vi "set 6221 level(SubVI).vi"(8 "错误输入（无错误）":errorcluster, 10 "电流（mA）":dbl, 11 "VISA引用句柄输入":refnum<visa-resource-name>) -> (0 "错误输出":errorcluster, 3 "VISA引用句柄输出":refnum<visa-resource-name>)   [LabVIEW 2019, in "SubVI.lvlib"]
uses:
  SubVI.lvlib
  lib/Keithley 622x/Configure/Delta PDelta DCon Modes/Low Level/Typedefs/KE622x -- Delta PDelta Mode High Level.ctl
  lib/Keithley 622x/Keithley 622x.lvlib
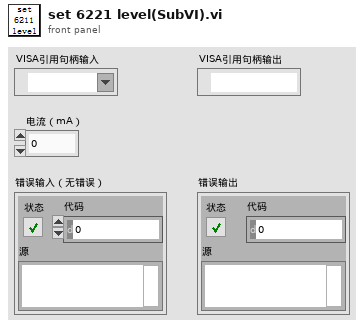
[diagram p1: front panel]
types:
  T1 = typedef "Keithley 622x.lvlib/KE622x -- Delta PDelta Mode High Level.ctl" = dbl
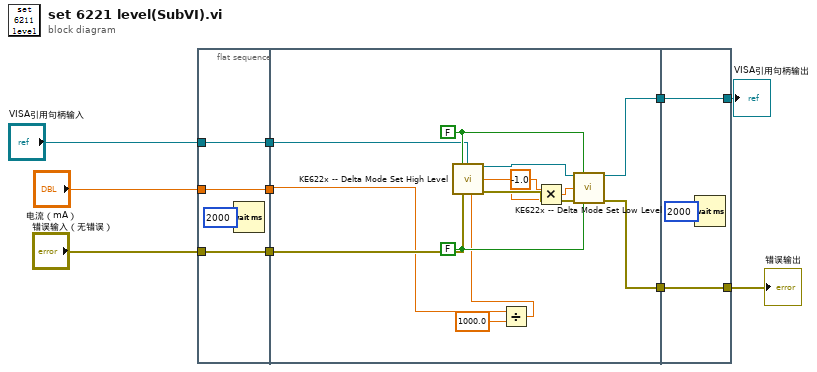
[diagram p0: block diagram]
diagram:
  n1 = flat-sequence {
    tunnel: "电流（mA）" -> [w12]
    tunnel: "VISA引用句柄输入" -> [w13]
    tunnel: "错误输入（无错误）" -> [w14]
    tunnel: [w14] -> w5
    tunnel: [w13] -> w4
    tunnel: [w12] -> w3
    tunnel: w5 -> [w28]
    tunnel: w4 -> [w22]
    tunnel: w3 -> [w17]
    tunnel: [w25] -> w2
    tunnel: [w23] -> w1
    tunnel: [w30] -> w8
    tunnel: [w31] -> w9
    tunnel: w2 -> [w31]
    tunnel: w1 -> [w30]
    frame #0 {
      n2 = Wait (ms)(milliseconds to wait=u32 2000) -> ()  [unwired: 1 out]
    }
    frame #1 {
      w27 = FALSE
      w26 = FALSE ("Check For SCPI Errors? (T)")
      n3 = Divide(x=w17, y=1000.0) -> (x/y=w16:dbl)
      n4 = call "KE622x -- Delta Mode Set High Level.vi"("Resource In"=w22, "Check For SCPI Errors? (T)"=w26, "High Level In (A)"=w16, "error in (no error)"=w28, "Read Back Set Value? (T)"=w27) -> ("Resource Out (dupl)"=w18:refnum<visa-resource-name>, "High Level Out (A)"=w19:T1, "error out"=w24:errorcluster)  [unwired: 8 in]
      n5 = Multiply(x=T1 -1.0, y=w19) -> (x*y=w21:T1)
      n6 = call "KE622x -- Delta Mode Set Low Level.vi"("Resource In"=w18, "Check For SCPI Errors? (T)"=w26, "Low Level In (A)"=w21, "error in (no error)"=w24, "Read Back Set Value? (T)"=w27) -> ("Resource Out (dupl)"=w23:refnum<visa-resource-name>, "error out"=w25:errorcluster)  [unwired: 8 in, 1 out]
    }
    frame #2 {
      n7 = Wait (ms)(milliseconds to wait=u32 2000) -> ()  [unwired: 1 out]
    }
  }
  "错误输出" <- w9
  "VISA引用句柄输出" <- w8
